vi "Clear Spy Queue.vi"(8 "error in (no error)":errorcluster, 11 "Mock Process In":refnum<class "Mock Error Handler.lvclass">) -> (0 "error out":errorcluster, 3 "Mock Process Out":refnum<class "Mock Error Handler.lvclass">)   [LabVIEW 2020, in "Mock Error Handler.lvclass"]
doc: "Clears any resorces allocated during initialization."
uses:
  Mock Error Handler.lvclass
  Mock Error Handler.lvclass/Mock Error Handler.ctl
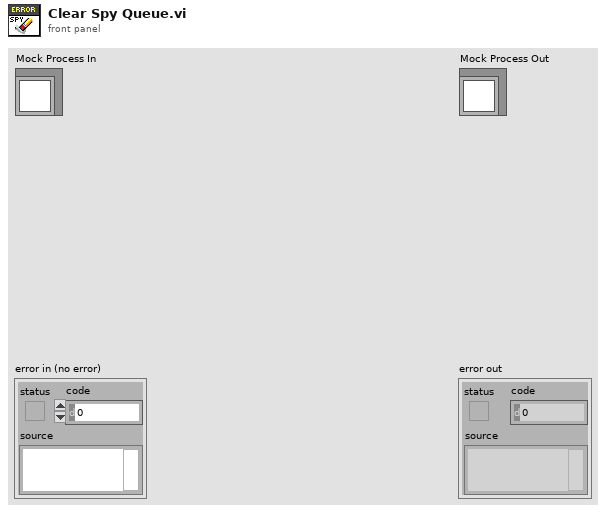
[diagram p1: front panel]
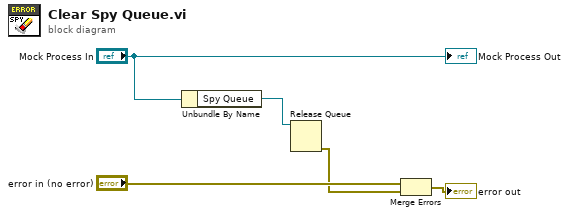
[diagram p0: block diagram]
diagram:
  n1 = Unbundle By Name("Mock Process In") -> ("Spy Queue"=w2:refnum<queue>)
  n2 = Release Queue(queue=w2) -> (error out=w1:errorcluster)  [unwired: 2 in, 2 out]
  n3 = Merge Errors("error in (no error)", w1) -> (→"error out":errorcluster)
  "Mock Process Out" <- "Mock Process In"
